vi "convert_double_to_string.vi"(4 "double in":dbl format="%#.12g", 5 "String to add before (\"\")":string) -> (1 "string out":string)   [LabVIEW 2022 SP3, in "hmp4000_rsidr_core.lvlib"]
uses:
  hmp4000_rsidr_core.lvlib
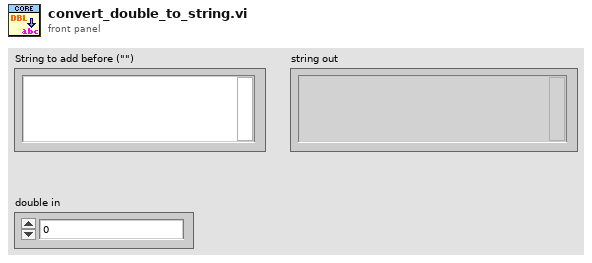
[diagram p1: front panel]
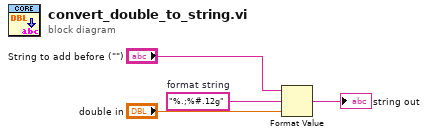
[diagram p0: block diagram]
diagram:
  w1 = "%.;%#.12g"  # format string
  n1 = Format Value(string ("")="String to add before (\"\")", format string=w1, value (0)="double in") -> (output string=→"string out":string)
